vi "Relink Maps to Entries.vi"(8 "error in (no error)":errorcluster, 11 "LV-Protoc in":refnum<class "LV-Protoc.lvclass">) -> (0 "error out":errorcluster, 3 "LV-Protoc out":refnum<class "LV-Protoc.lvclass">)   [LabVIEW 2020, in "LV-Protoc.lvlib" / "LV-Protoc.lvclass"]
doc: "Replaces map fields with a nested repeated message field for their actual implementation."
uses:
  LV-Protoc.lvclass
  LV-Protoc.lvclass/LV-Protoc.ctl
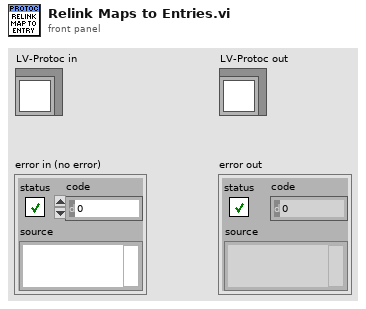
[diagram p1: front panel]
types:
  T1 = typedef "LV-Proto.lvlib/Message.ctl" = cluster{"Name":string, "Fields":T2[], "Reserved Numbers":u32[], "Reserved Names":string[]}
  T2 = typedef "LV-Proto.lvlib/Field.ctl" = cluster{"Name":string, "Number":u32, "Optional":bool, "Repeated":bool, "Type":T3, "Key Type":T3, "Value Type":T3}
  T3 = typedef "LV-Proto.lvlib/Type.ctl" = cluster{"Type":T4, "Subtype":string}
  T4 = typedef "LV-Proto.lvlib/Proto Type.ctl" = enum16{"UNKNOWN", "double", "float", "int32", "int64", "uint32", "uint64", "sint32", "sint64", "fixed32", "fixed64", "sfixed32", "sfixed64", "bool", "string", "bytes", "enum", "map", "message"}
  T5 = typedef "LV-Protoc.lvlib/Map Typenames.ctl" = cluster{"Entry":string, "Key":string, "Value":string}
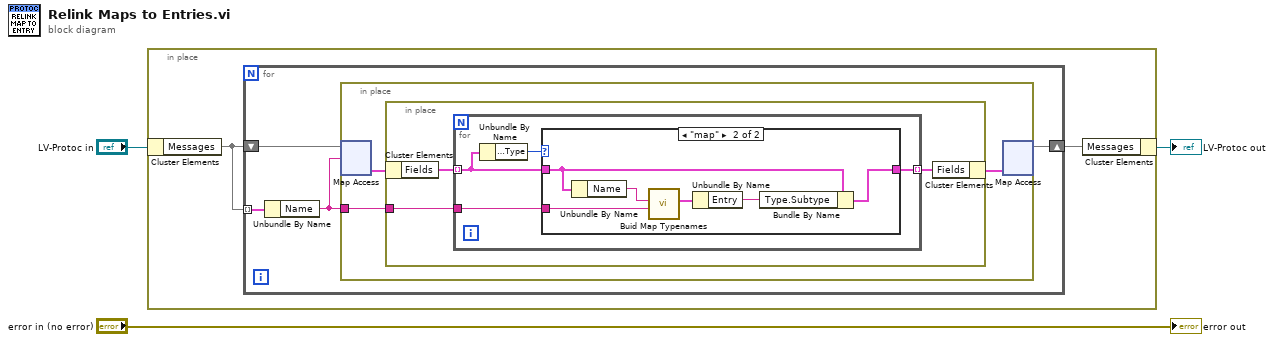
[diagram p0: block diagram]
diagram:
  n1 = in-place {
    n2 = in-place-cluster #1("LV-Protoc in") -> ("Messages"=w5:map{string, T1})
    n3 = for {
      tunnel: w5 -> [w9] mode=indexing
      shift-right: [w7] -> w4
      shift-left: w5 -> [w8]
      n4 = Unbundle By Name(w9) -> ("Name"=w6:string)
      n5 = in-place {
        in-place-border: w6 -> [w10]
        n6 = in-place-map #2(w8, w6) -> (w11:T1)  [unwired: 1 in, 1 out]
        n7 = in-place {
          in-place-border: w10 -> [w13]
          n8 = in-place-cluster #3(w11) -> ("Fields"=w15:T2[])
          n9 = for {
            tunnel: w15 -> [w18] mode=indexing
            tunnel: [w17] -> w14 mode=indexing
            tunnel: w13 -> [w16]
            n10 = Unbundle By Name(w18) -> ("Type.Type"=w19:T4)
            n11 = case shown="\"map\"" w19 {
              tunnel: w18 -> [w20 w22]
              tunnel: [w20 w23] -> w17
              tunnel: w16 -> [_ w25]
              frame Default {
              }
              frame "map" {
                n12 = Unbundle By Name(w22) -> ("Name"=w21:string)
                n13 = call "Buid Map Typenames.vi"("Message Name"=w25, "Map Name"=w21) -> ("Map Typenames"=w26:T5)  [unwired: 8 in, 1 out]
                n14 = Unbundle By Name(w26) -> ("Entry"=w24:string)
                n15 = Bundle By Name(cluster=w22, "Type.Subtype"=w24) -> (w23:T2)
              }
            }
          }
          n16 = in-place-cluster #3("Fields"=w14) -> (w12:T1)
        }
        n17 = in-place-map #2(w12) -> (w7:map{string, T1})  [unwired: 1 in, 2 out]
      }
    }
    n18 = in-place-cluster #1("Messages"=w4) -> (→"LV-Protoc out":refnum<class "LV-Protoc.lvclass">)
  }
  "error out" <- "error in (no error)"
